vi "Config.vi"(8 "error in (no error)":errorcluster, 9 "Action":enum16{"Read", "Write"}(ring), 10 "Variable Name":string, 11 "Variable Value In":variant) -> (0 "error out":errorcluster, 3 "Variable Value Out":variant)   [LabVIEW 2018, in "Main.lvlib"]
uses:
  Main.lvlib
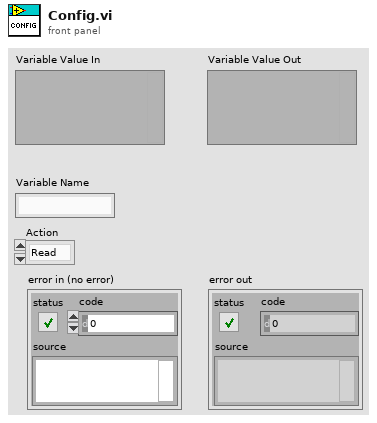
[diagram p1: front panel]
types:
  T1 = enum32{"invalid app kind", "Development System", "Run Time System", "Student Edition", "Embedded LabVIEW", "Evaluation", "Custom"}
  T2 = cluster{"DAQ":tag, "Primary Mixer":tag, "Primary Screw":tag, "Primary Solenoid":tag, "Inner Flow":refnum<visa-resource-name>, "Outer Flow":refnum<visa-resource-name>, "Chamber Pressure":tag, "Feeder Pressure":tag, "Stage":refnum<visa-resource-name>}
  T3 = cluster{"Screw":u16, "Inner":dbl, "Outer":dbl, "Mixer":dbl}
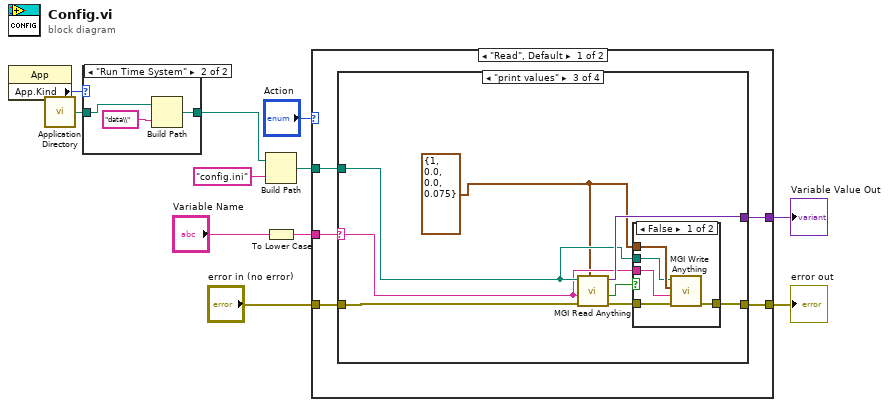
[diagram p0: block diagram]
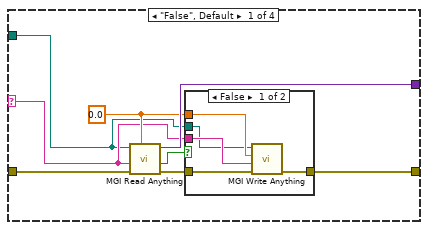
[diagram p3: hidden frame]
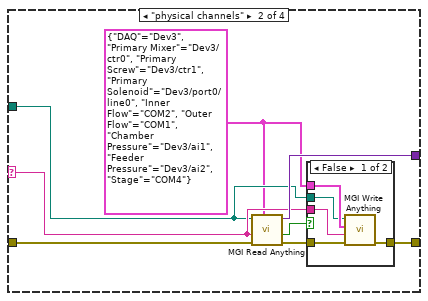
[diagram p5: hidden frame]
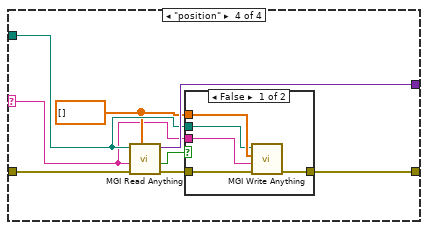
[diagram p8: hidden frame]
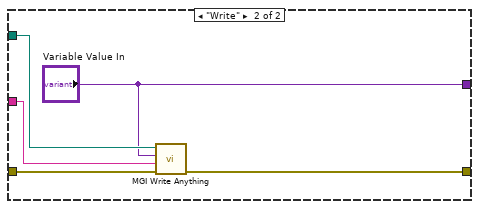
[diagram p10: hidden frame]
diagram:
  n1 = property class="App"() -> ("App.Kind"=w10:T1)  [unwired: 2 in, 2 out]
  n2 = call <vilib>:"Application Directory.vi"() -> ("Application Directory"=w9:path)
  n3 = case shown="\"Run Time System\"" w10 {
    tunnel: w9 -> [w12 w15]
    tunnel: [w12 w14] -> w8
    frame "Development System", Default {
    }
    frame "Run Time System" {
      n4 = Build Path(base path=w15, name or relative path="data\\") -> (appended path=w14:path)
    }
  }
  n5 = Build Path(base path=w8, name or relative path="config.ini") -> (appended path=w4:path)
  n6 = To Lower Case(string="Variable Name") -> (all lower case string=w1:string)
  n7 = case shown="\"Read\", Default" "Action" {
    tunnel: w1 -> [w19 w81]
    tunnel: [w16 "Variable Value In"] -> w5
    tunnel: w4 -> [w18 w80]
    tunnel: [w17 w77] -> w3
    tunnel: "error in (no error)" -> [w20 w78]
    frame "Read", Default {
      n8 = case shown="\"print values\"" w19 {
        selector: w19 -> [w23 w38 w50 w63]
        tunnel: w20 -> [w28 w42 w52 w70]
        tunnel: w18 -> [w22 w37 w51 w65]
        tunnel: [w25 w39 w53 w66] -> w17
        tunnel: [w27 w41 w54 w69] -> w16
        frame "False", Default {
          w24 = 0.0
          n9 = call <userlib>:"MGI Read Anything.vi"("Type of Anything"=w24, "Error In"=w28, "Section Name (Name of \"Type of Anything\")"=w23, "Path (dialog)"=w22) -> ("Error Out"=w26:errorcluster, "Found?"=w21:bool, "Anything"=w27:variant)  [unwired: 4 in, 1 out]
          n10 = case shown="False" w21 {
            tunnel: w26 -> [w33 w34]
            tunnel: [w29 w34] -> w25
            tunnel: w22 -> [w30 _]
            tunnel: w24 -> [w32 _]
            tunnel: w23 -> [w31 _]
            frame False {
              n11 = call <userlib>:"MGI Write Anything.vi"("Error In"=w33, "Section Name (Name of \"Anything\")"=w31, "Anything"=w32, "Path (dialog)"=w30) -> ("Error Out"=w29:errorcluster)  [unwired: 5 in, 2 out]
            }
            frame True {
            }
          }
        }
        frame "physical channels" {
          w35 = T2 {"DAQ"="Dev3", "Primary Mixer"="Dev3/ctr0", "Primary Screw"="Dev3/ctr1", "Primary Solenoid"="Dev3/port0/line0", "Inner Flow"="COM2", "Outer Flow"="COM1", "Chamber Pressure"="Dev3/ai1", "Feeder Pressure"="Dev3/ai2", "Stage"="COM4"} ("Physical Channels")
          n12 = call <userlib>:"MGI Read Anything.vi"("Type of Anything"=w35, "Error In"=w42, "Section Name (Name of \"Type of Anything\")"=w38, "Path (dialog)"=w37) -> ("Error Out"=w40:errorcluster, "Found?"=w36:bool, "Anything"=w41:variant)  [unwired: 4 in, 1 out]
          n13 = case shown="False" w36 {
            tunnel: w40 -> [w47 w48]
            tunnel: [w43 w48] -> w39
            tunnel: w37 -> [w44 _]
            tunnel: w35 -> [w46 _]
            tunnel: w38 -> [w45 _]
            frame False {
              n14 = call <userlib>:"MGI Write Anything.vi"("Error In"=w47, "Section Name (Name of \"Anything\")"=w45, "Anything"=w46, "Path (dialog)"=w44) -> ("Error Out"=w43:errorcluster)  [unwired: 5 in, 2 out]
            }
            frame True {
            }
          }
        }
        frame "print values" {
          w49 = T3 {"Screw"=1, "Inner"=0.0, "Outer"=0.0, "Mixer"=0.075} ("Print Values 2")
          n15 = call <userlib>:"MGI Read Anything.vi"("Type of Anything"=w49, "Error In"=w52, "Section Name (Name of \"Type of Anything\")"=w50, "Path (dialog)"=w51) -> ("Error Out"=w56:errorcluster, "Found?"=w55:bool, "Anything"=w54:variant)  [unwired: 4 in, 1 out]
          n16 = case shown="False" w55 {
            tunnel: w56 -> [w61 w62]
            tunnel: [w57 w62] -> w53
            tunnel: w51 -> [w58 _]
            tunnel: w49 -> [w60 _]
            tunnel: w50 -> [w59 _]
            frame False {
              n17 = call <userlib>:"MGI Write Anything.vi"("Error In"=w61, "Section Name (Name of \"Anything\")"=w59, "Anything"=w60, "Path (dialog)"=w58) -> ("Error Out"=w57:errorcluster)  [unwired: 5 in, 2 out]
            }
            frame True {
            }
          }
        }
        frame "position" {
          w64 = dbl[] []
          n18 = call <userlib>:"MGI Read Anything.vi"("Type of Anything"=w64, "Error In"=w70, "Section Name (Name of \"Type of Anything\")"=w63, "Path (dialog)"=w65) -> ("Error Out"=w68:errorcluster, "Found?"=w67:bool, "Anything"=w69:variant)  [unwired: 4 in, 1 out]
          n19 = case shown="False" w67 {
            tunnel: w68 -> [w75 w76]
            tunnel: [w71 w76] -> w66
            tunnel: w65 -> [w72 _]
            tunnel: w64 -> [w74 _]
            tunnel: w63 -> [w73 _]
            frame False {
              n20 = call <userlib>:"MGI Write Anything.vi"("Error In"=w75, "Section Name (Name of \"Anything\")"=w73, "Anything"=w74, "Path (dialog)"=w72) -> ("Error Out"=w71:errorcluster)  [unwired: 5 in, 2 out]
            }
            frame True {
            }
          }
        }
      }
    }
    frame "Write" {
      n21 = call <userlib>:"MGI Write Anything.vi"("Error In"=w78, "Section Name (Name of \"Anything\")"=w81, "Anything"="Variable Value In", "Path (dialog)"=w80) -> ("Error Out"=w77:errorcluster)  [unwired: 5 in, 2 out]
    }
  }
  "error out" <- w3
  "Variable Value Out" <- w5
